vi "DB Tools Save Recordset To File.vi"   [LabVIEW 2020, in "NI_Database_API.lvlib"]
doc: "Saves the recordset identified by the <B>recordset reference</B> to either an XML or ADTG file. The ADTG file format is a proprietary format that only the LabVIEW Database Connectivity Toolkit can interpret. The ADTG format results in a smaller file than the XML format. You can reload both formats into LabVIEW using the DB Tools Load Recordset From File VI.\n\nWire data to the reference input to determine the polymorphic instance to use or manually select the instance."
uses:
  <vilib>/addons/database/NI_Database_API.lvlib
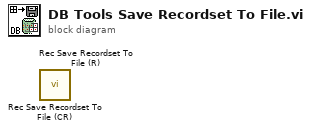
[diagram p0: block diagram]
diagram:
  n1 = call <vilib>:"Rec Save Recordset To File (CR).vi"() -> ()  [unwired: 8 in, 2 out]
  n2 = call <vilib>:"Rec Save Recordset To File (R).vi"() -> ()  [unwired: 8 in, 2 out]
